vi "PAN_AddModule.vi"(8 "Mods in":string[](array[string]), 9 "Translations In":string[][](array[string]), 10 "modpath":path, 11 "module name":string) -> (0 "Mods Out":string[](array[string]), 1 "Translations out":string[][](array[string]))   [LabVIEW 2016]
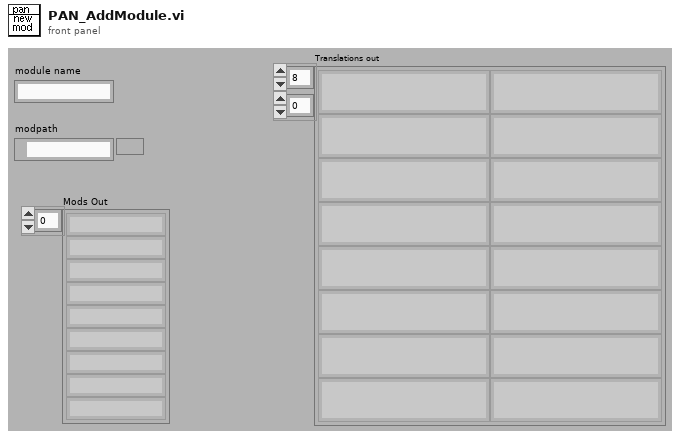
[diagram p1: front panel]
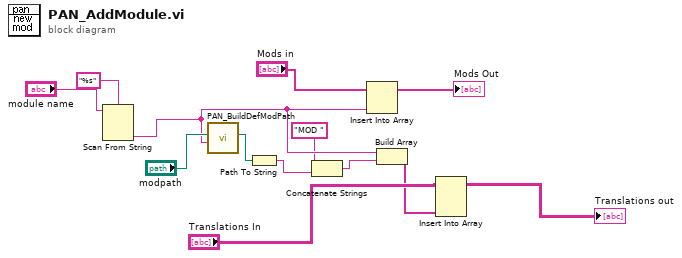
[diagram p0: block diagram]
diagram:
  n1 = Scan From String(format string="%s", input string="module name") -> (output 1=w4:string)  [unwired: 2 in, 4 out]
  n2 = call "PAN_BuildDefModPath.vi"("mod name"=w4, "modpath"="modpath") -> ("modapipath"=w7:path)  [unwired: 9 out]
  n3 = Path To String(path=w7) -> (string=w3:string)
  n4 = Concatenate Strings("MOD " ("string"), w3) -> (w1:string)
  n5 = Insert Into Array(array="Mods in", new element=w4) -> (→"Mods Out":string[])  [unwired: 1 in]
  n6 = Build Array(w4, w1) -> (w9:string[])
  n7 = Insert Into Array(array="Translations In", new element=w9) -> (→"Translations out":string[][])  [unwired: 2 in]
